vi "TRITON_Set field and rate.vi"(1 "target field":dbl format="%#_13g", 2 "error in (no error)":errorcluster, 3 "Sweep rate":dbl=0.1) -> (0 "error out":errorcluster)   [LabVIEW 2021]
panel:
  out "Response String":string
  in  "Mode":T1(ring)=enum."Immediate"
  in  "Bytes to Read":i32=5000
  in  "IP Address":string="192.168.0.2"
  in  "Remote Port":i32=33576
  in  "Timeout":i32=10000
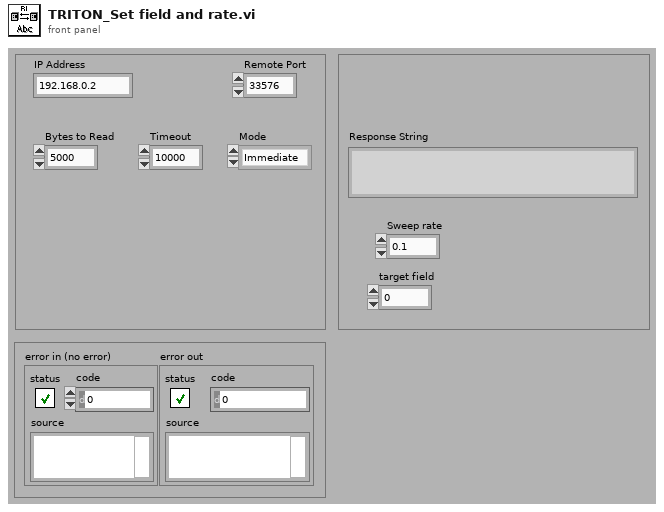
[diagram p1: front panel]
types:
  T1 = enum16{"Standard", "Buffered", "CRLF", "Immediate"}
  T2 = cluster{"Mode":enum16{"Standard", "Buffered", "CRLF", "Immediate"}, "Bytes to Read":i32, "IP Address":string, "Remote Port":i32, "Timeout":i32}
  T3 = cluster{"Mode":enum16{"Standard", "Buffered", "CRLF", "Immediate"}, "Bytes to Read":i32, "IP Address":string, "Remote Port":i32, "Timeout":i32, "connection ID":refnum<k5>}
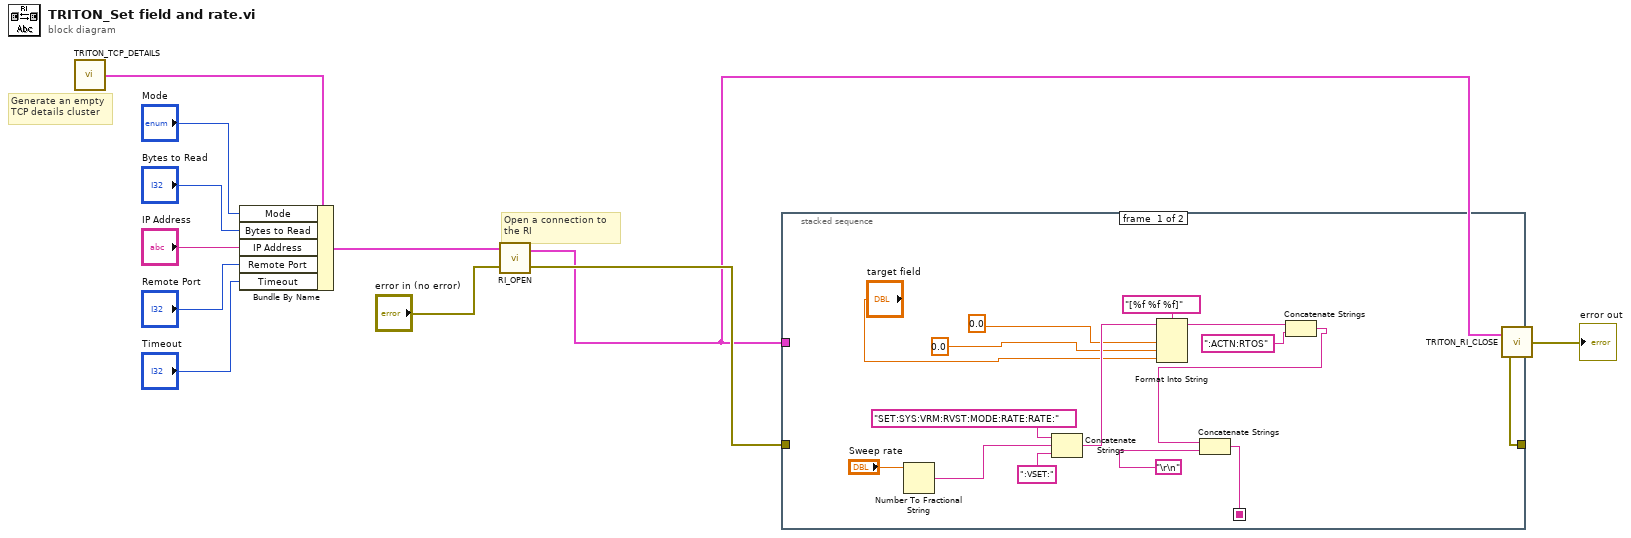
[diagram p0: block diagram]
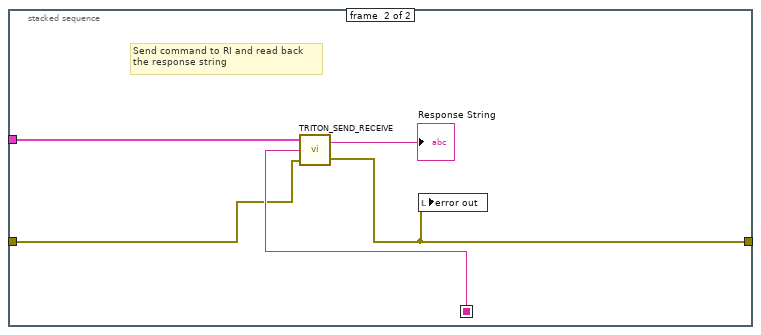
[diagram p2: hidden frame]
diagram:
  # "Open a connection to\nthe RI"
  # "Generate an empty\nTCP details cluster"
  n1 = call "TRITON_TCP_DETAILS.vi"() -> ("Cluster"=w12:T2)
  n2 = Bundle By Name(cluster=w12, "Mode"="Mode", "Bytes to Read"="Bytes to Read", "IP Address"="IP Address", "Remote Port"="Remote Port", "Timeout"="Timeout") -> (w10:T2)
  n3 = call "RI_OPEN.vi"("error in (no error)"="error in (no error)", "Cluster"=w10) -> ("error out"=w9:errorcluster, "output cluster"=w6:T3)
  n4 = stacked-sequence {
    seq-local: [w26 _] -> [_ w31]
    tunnel: w9 -> [_ w30]
    tunnel: [_ w29] -> w8
    tunnel: w6 -> [_ w28]
    frame #0 {
      n5 = Number To Fractional String(number="Sweep rate") -> (F-format string=w18:string)  [unwired: 3 in]
      n6 = Concatenate Strings("SET:SYS:VRM:RVST:MODE:RATE:RATE:", w18, ":VSET:") -> (w17:string)
      n7 = Format Into String(format string="[%f %f %f]", initial string=w17, 0.0, 0.0, "target field") -> (resulting string=w23:string)  [unwired: 1 in, 1 out]
      n8 = Concatenate Strings(w23, ":ACTN:RTOS") -> (w13:string)
      n9 = Concatenate Strings(w13, "\r\n") -> (w26:string)
    }
    frame #1 {
      # "Send command to RI and read back\nthe response string"
      n10 = call "TRITON_SEND_RECEIVE.vi"("error in (no error)"=w30, "Command String"=w31, "Communication Cluster"=w28) -> ("error out"=w29:errorcluster, "Response String"=→"Response String":string)
      n11 = local write "error out"(w29) -> ()
    }
  }
  n12 = call "TRITON_RI_CLOSE.vi"("error in (no error)"=w8, "Communication Cluster"=w6) -> ("error out"=→"error out":errorcluster)
